vi "Samwontech TEMP2xxx Driver Test.vi"() -> ()   [LabVIEW 2017]
uses:
  <instrlib>/Samwontech TEMP2xxx/Samwontech TEMP2xxx.lvlib
panel:
  out "Checksum":string
  out "Command":string
  out "Address":string
  out "Value (decimal)":u32
  out "Value (string)":string
  out "OK":string
  out "STX":string
  in  "Responce":string="\u000201RSD,OK,01F405"
  out "Request":string
  in  "Checksum":bool=TRUE
  in  "D-register number":u8=5
  in  "Count number":u8=1
  in  "Address":u8=1
  # "RSD Command Compose"
  # "RSD Command Parse"
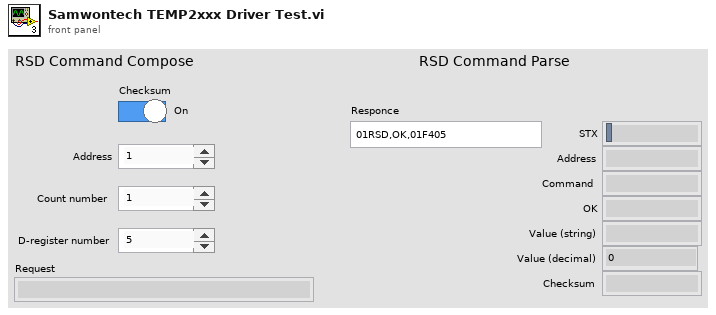
[diagram p1: front panel]
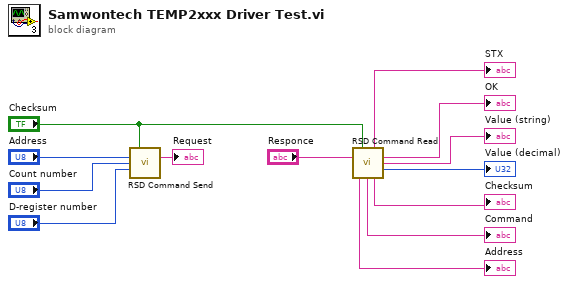
[diagram p0: block diagram]
diagram:
  n1 = call <instrlib>:"RSD Command Send.vi"("Checksum used"="Checksum", "Address"="Address", "Count number"="Count number", "D-register number"="D-register number") -> ("Request"=→"Request":string)  [unwired: 9 in, 2 out]
  n2 = call <instrlib>:"RSD Command Read.vi"("Checksum used"="Checksum", "Responce"="Responce") -> ("STX"=→"STX":string, "OK"=→"OK":string, "Value (string)"=→"Value (string)":string, "Value (decimal)"=→"Value (decimal)":u32, "Address"=→"Address":string, "Command"=→"Command":string, "Checksum"=→"Checksum":string)  [unwired: 5 in, 2 out]
